vi "Topo & GridSpectr_DriftCorrection_zSpec_v15.vi"(6 "Internal use":string, 7 "Grid param":T1 {"height (m)" format="%#_6p"; "width (m)" format="%#_6p"; "center Y (m)" format="%#_6p"; "center X (m)" format="%#_6p"}, 8 "Error in (no error)":errorcluster, 9 "Points Y/Index Y":i32, 10 "Points X/Index X":i32, 11 "Method":enum16{"init", "run", "end"}(ring)=enum."end") -> (0 "Error out":errorcluster)   [LabVIEW 2014]
doc: "Example of a measurement VI to be used in the \"Experiments on a Grid\" tool as external VI.\n\nThis example measure the topography and spectroscopy data. The spectroscopy measurements are taken on a subgrid. The data are saved to a sxm and a binary file.\n\n- Nanonis Programming Interface -"
uses:
  <userlib>/Nanonis Prog Interface V5/Scan/Grid/GridPatternGet.vi
  <userlib>/Nanonis Prog Interface V5/Scan/Grid/LinePatternGet.vi
  <userlib>/Nanonis Prog Interface V5/Nanonis Prog Interface.lvlib
panel:
  in  "trigger 2 >Hz":sgl format="%#_6p"
  in  "trigger1 < Hz":sgl format="%#_6p"
  out "zFile":refnum<file>
  out "last z adjustment":sgl format="%#_6p"
  in  "during Spec Bias (V)":sgl format="%#_5p"
  in  "type":u16(ring)=1 items=["Line", "Grid"]
  in  "readjust setpoint every":i32=4
  in  "Correct Drift":bool=TRUE
  in  "Email when finished":string="cornelius.krull@monash.edu"
  in  "STS z offset":dbl format="%#_6p"
  out "ETA":timestamp
  out "remaining":dbl format="%<%H:%M:%S>t"
  out "Progress":u8(slide) scale=0.0..100.0 scale format="%#.1g"
  out "total Points":i32
  in  "preSTS delay [ms]":u32=500
  in  "ref Bias":dbl=0.02 format="%#_6p"
  in  "Imaging Bias":dbl=0.02 format="%#_6p"
  in  "max applied Drift Correction":i32=20 min=1 max=100 step=1 format="%.0p"
  in  "Correlate":u16(ring) items=["first Frame", "successive Frames"]
  out "Topo Images taken":i32=14
  in  "Increment":i32=40
  in  "Threshold":i32=2 min=1 step=1
  in  "tip Speed (m/s)":sgl=2e-09 format="%.2p"
  out "X drift":i32
  out "Y drift":i32
  out "Last Drift detected":i32=40
  in  "MaxImagesBack":i32=40
  in  "Channel index (0-23)":u8(ring) items=["Current"=0, "Z (m)"=14]
  in  "File name":string="symmetric_node"
  in  "ref Current":dbl=5e-12 format="%#_6p"
  in  "Imaging Current":dbl=5e-12 format="%#_6p"
  in  "zdrift \nDuration (s)":dbl
  in  "Correct z drift":bool
  out "Status":string="finishing"
  in  "Drift correction Pixels":i32=256 caption="Topo Pixels"
  out "Y Offset":dbl format="%#_6p"
  out "X Offset":dbl format="%#_6p"
  out "Points taken":dbl=14.0
  in  "Drift Correction every":i32=40
  in  "Y subgrid spacing":u16=1
  in  "X subgrid spacing":u16=1
  # "z Spectroscopy"
  # "GRID points"
  # "Increase this if no Drift was detected for \na certain number of images"
  # "%"
  # "time (HH:MM:SS)"
  # "images back"
  # "% of image size"
  # "RUN smart tilt before starting the GRID\nImg Angle = 0\nmove tip to reference point for tip height"
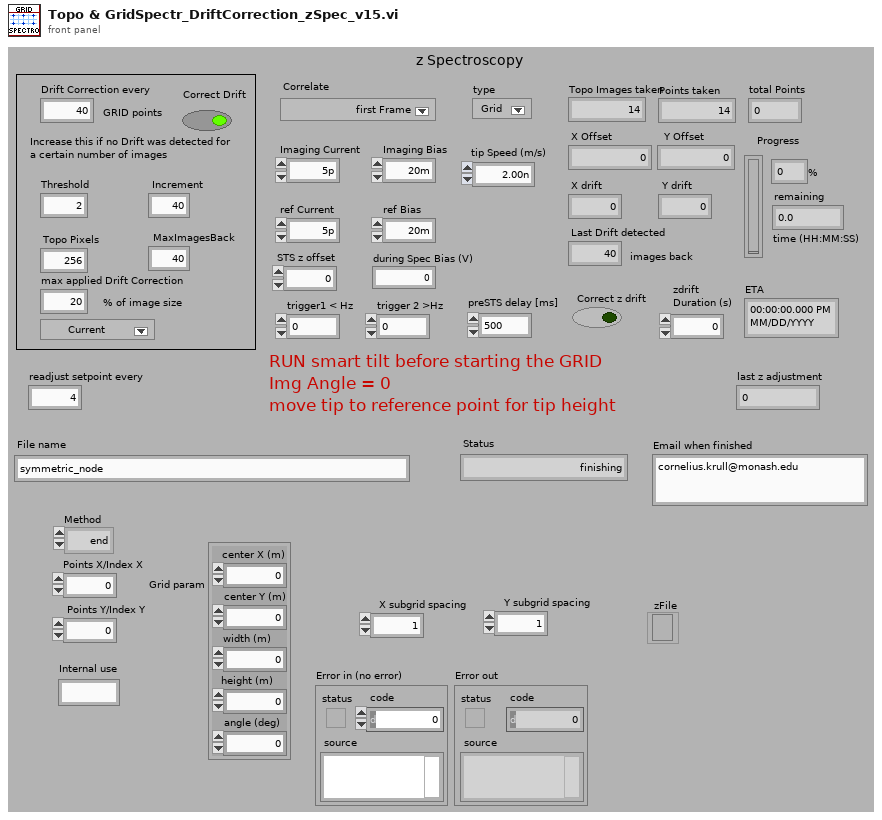
[diagram p1: front panel]
types:
  T1 = cluster{"center X (m)":sgl, "center Y (m)":sgl, "width (m)":sgl, "height (m)":sgl, "angle (deg)":sgl}
  T2 = enum16{"open", "replace", "create", "open or create", "replace or create", "replace or create with confirmation"}
  T3 = cluster{"Z averaging time (s)":sgl, "Z offset (m)":sgl, "Initial settling time (s)":sgl}
  T4 = cluster{"Drift correction Pixels":i32, "Imaging Current":dbl, "STS Current":dbl, "MaxImagesBack":i32, "tip Speed (m/s)":sgl, "Threshold":i32, "Increment":i32, "Correlate":u16, "max applied Drift Correction":i32, "Imaging Bias":dbl, "Move Current":dbl, "Move Bias":dbl, "STS Bias":dbl, "preSTS delay [ms]":u32, "STS z offset":dbl, "Correct Drift":bool, "Lockin ON/OFF":bool}
  T5 = cluster{"center X":sgl, "center Y":sgl, "angle":sgl, "width":sgl, "height":sgl, "# pixels":i32, "# lines":i32}
  T6 = cluster{"Name":string, "Calibration":sgl, "Offset":sgl, "Channel index":i32}[]
  T7 = cluster{"up/down":bool, "time/line":sgl, "start time":timestamp, "end time":timestamp}
  T8 = cluster{"Z averaging time (s)":sgl, "Initial settling time (s)":sgl}
  T9 = cluster{"Max. slew rate (m/s)":sgl, "Settling time (s)":sgl, "Integration time (s)":sgl}
  T10 = cluster{"End settling time (s)":sgl, "Z control time (s)":sgl}
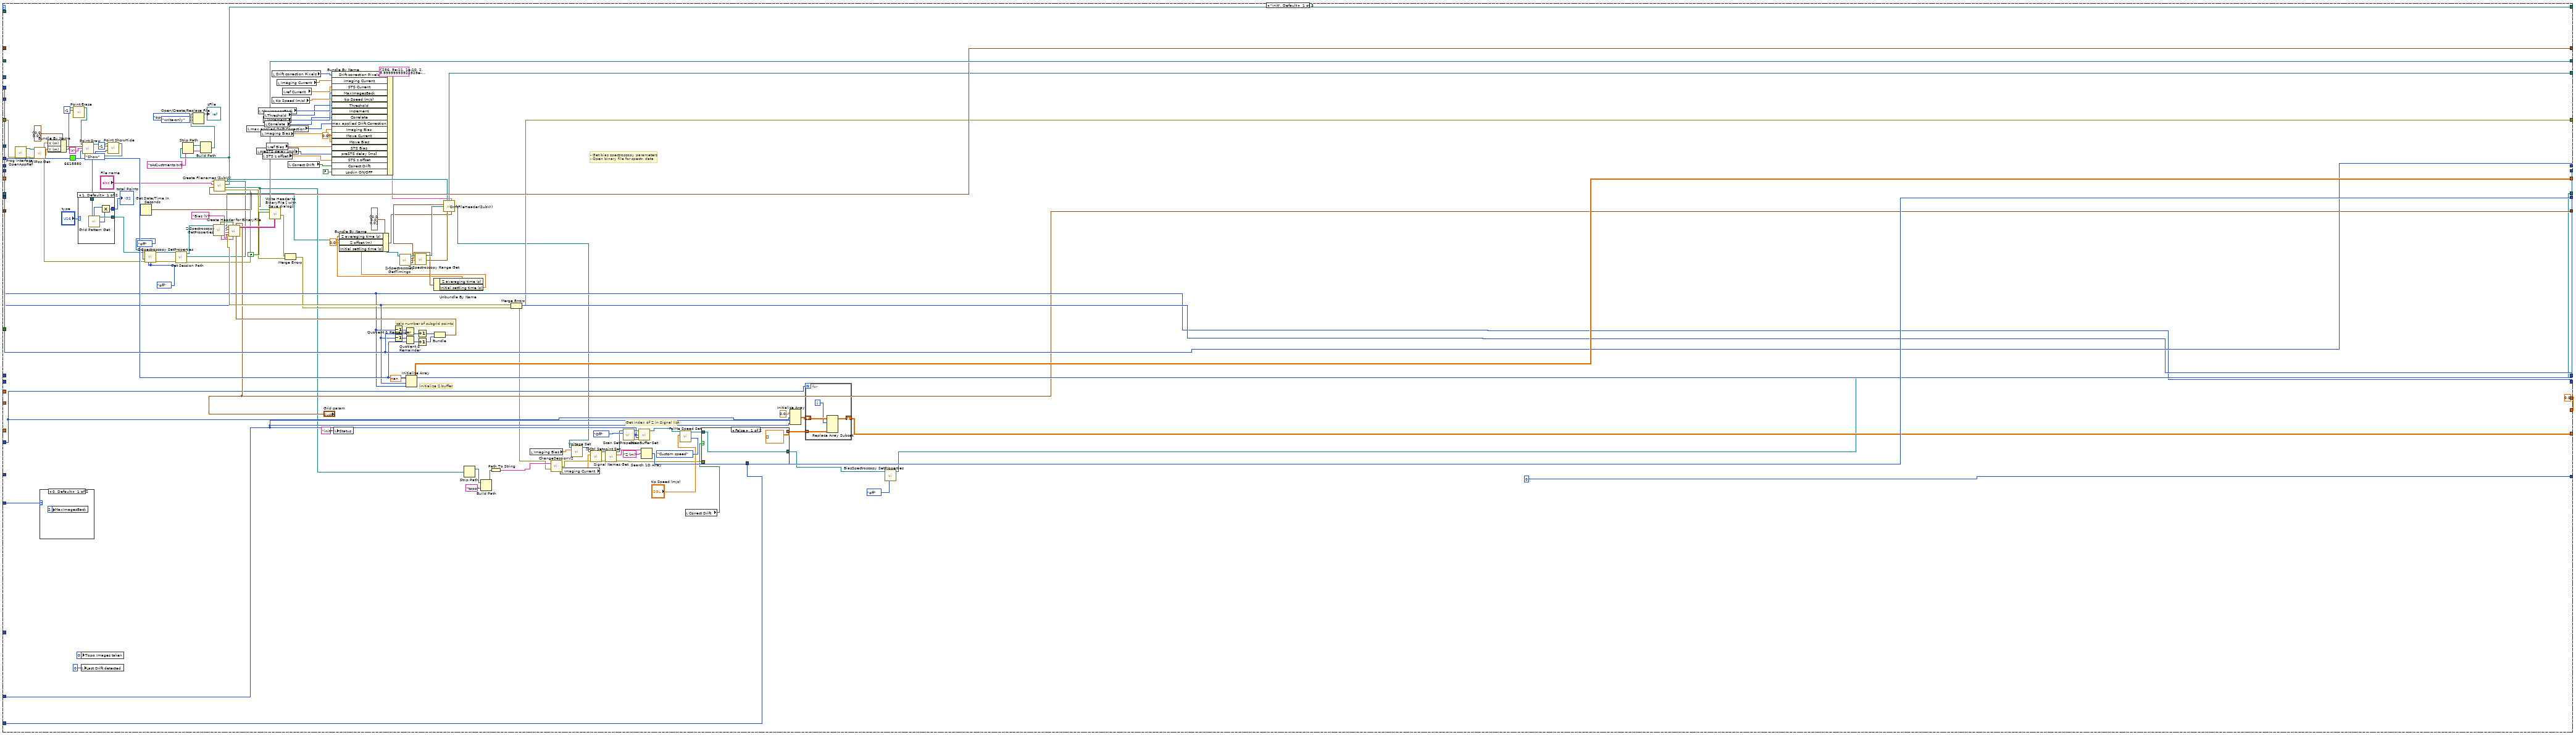
[diagram p2: hidden frame]
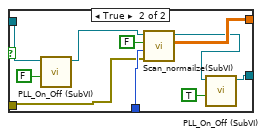
[diagram p3: hidden frame]
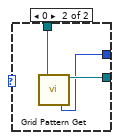
[diagram p4: hidden frame]
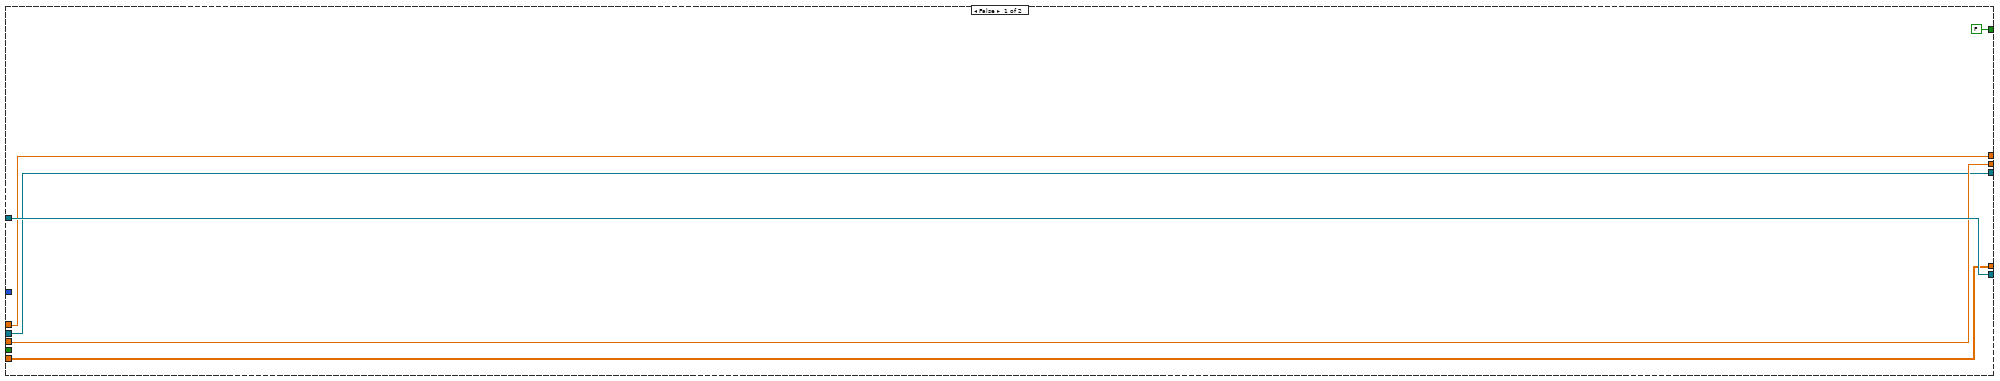
[diagram p9: hidden frame]
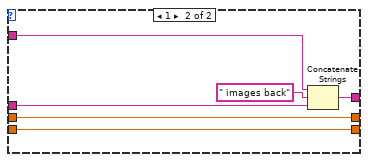
[diagram p10: hidden frame]
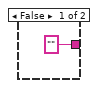
[diagram p12: hidden frame]
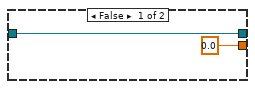
[diagram p13: hidden frame]
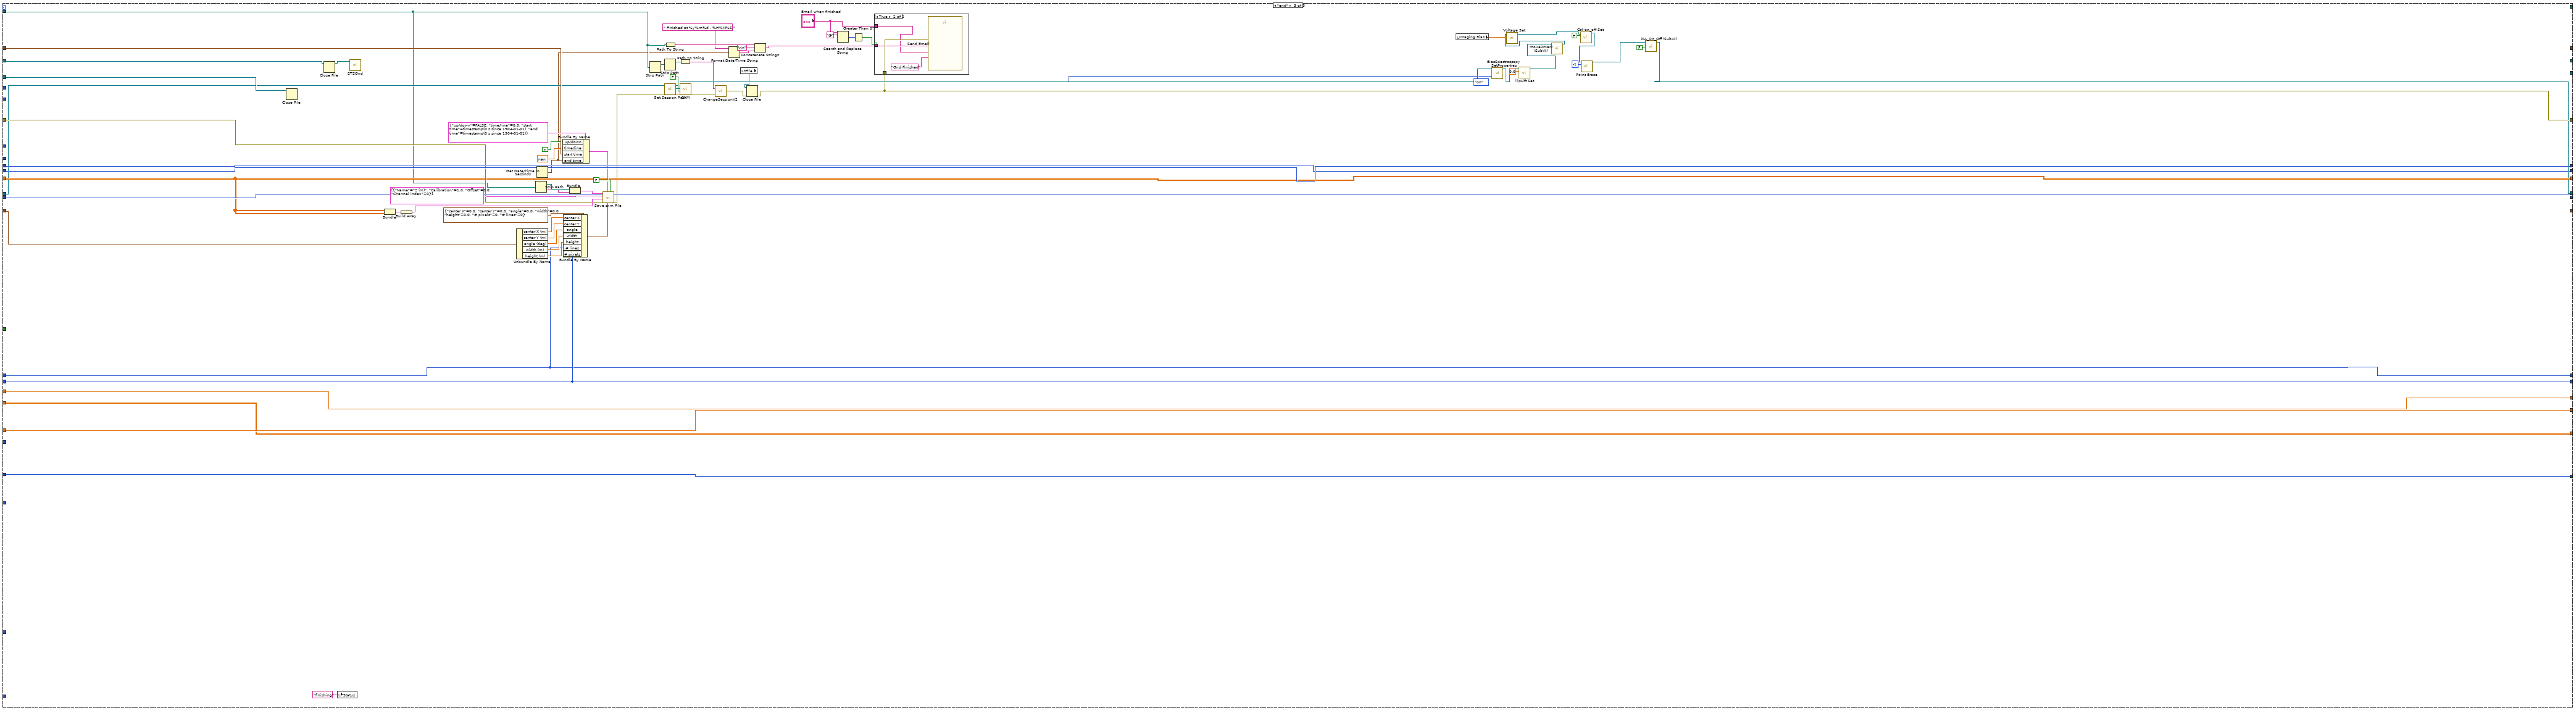
[diagram p15: hidden frame]
diagram:
  # "This string control is required so this VI's connector is compatible with the Nanonis module : \"Experiment on a grid\"."
  # "IMPORTANT : The connector of your own VI must EXACTLY match the connector of this example VI.\n\nThis example VI will do the following:\n- init: Open/Create a sxm (scan data file). Store file path in shift register. Initialize buffer for the topography data. Open binary file and create header.\n- run: Get Z position and write it to topography buffer (from last row to first row of buffer, to make it compatible to Save sxm File function which assumes data starting on the top left corner of image). If grid indices x,y are multiples of the subgrid spacings, start a bias spectroscopy experiment. Write the spectroscopy data to the binary file.\n- end: Write data from topography buffer to file, along with grid dimensions and other known parameters. Close files."
  n1 = while {
    shift-right: [w21] -> _
    shift-left: _ -> [w44]
    shift-right: [w39] -> _
    shift-left: _ -> [w38]
    shift-right: [w36] -> _
    shift-left: _ -> [w37]
    shift-right: [w35] -> _
    shift-left: _ -> [w34]
    shift-right: [w28] -> _
    shift-left: _ -> [w30]
    shift-right: [w29] -> _
    shift-left: _ -> [w31]
    shift-right: [w27] -> _
    shift-left: _ -> [w26]
    shift-right: [w25] -> _
    shift-left: _ -> [w24]
    shift-right: [w23] -> _
    shift-left: _ -> [w22]
    shift-right: [w20] -> _
    shift-left: _ -> [w19]
    shift-right: [w18] -> _
    shift-left: _ -> [w17]
    shift-right: [w16] -> _
    shift-left: _ -> [w9]
    shift-right: [w15] -> _
    shift-left: _ -> [w8]
    shift-right: [w14] -> _
    shift-left: _ -> [w11]
    shift-right: [w13] -> _
    shift-left: _ -> [w10]
    shift-right: [w6] -> _
    shift-left: _ -> [w5]
    stop <- TRUE stop-if-true
    # "> Drift file ref >"
    # "> number of  points  >"
    # "> Ref Frame  >"
    # "> Grid param >"
    # "> start time >"
    # ">Application reference >"
    # "> Y Subgrid spacing >"
    # "> X Subgrid spacing >"
    # "> Z signal index >"
    # "> Binary file ref >"
    # "> Z buffer >"
    # "> sxm file path >"
    n2 = case shown="\"run\"" "Method" {
      tunnel: [w53 w279 _] -> w21
      tunnel: w44 -> [_ w279 w485]
      tunnel: "Error in (no error)" -> [w147 w265 w515]
      tunnel: [w127 w278 w462] -> w42
      tunnel: "Points X/Index X" -> [w159 w273 _]
      tunnel: "Points Y/Index Y" -> [w160 w259 _]
      tunnel: [w183 w276 w504] -> w39
      tunnel: w38 -> [_ w277 w504]
      tunnel: w37 -> [_ w275 w497]
      tunnel: [w175 w274 _] -> w36
      tunnel: [w173 w209 w529] -> w35
      tunnel: w34 -> [_ w209 w529]
      tunnel: "X subgrid spacing" -> [w172 _ _]
      tunnel: "Y subgrid spacing" -> [w171 _ _]
      tunnel: w31 -> [_ w267 w528]
      tunnel: w30 -> [_ w266 w527]
      tunnel: [w172 w267 w528] -> w29
      tunnel: [w171 w266 w527] -> w28
      tunnel: [w112 w252 w460] -> w27
      tunnel: w26 -> [_ w236 w490]
      tunnel: ["Grid param" w262 _] -> w25
      tunnel: w24 -> [_ w262 w514]
      tunnel: [w145 w227 _] -> w23
      tunnel: w22 -> [_ w227 w522]
      tunnel: [w160 w260 w505] -> w20
      tunnel: w19 -> [_ w260 w505]
      tunnel: [w159 w261 w506] -> w18
      tunnel: w17 -> [_ w261 w506]
      tunnel: [w156 w242 w503] -> w16
      tunnel: [w156 w247 w501] -> w15
      tunnel: [w141 w241 w498] -> w14
      tunnel: [0 w225 w502] -> w13
      tunnel: w10 -> [_ w211 w502]
      tunnel: "Drift Correction every" -> [_ w255 _]
      tunnel: w11 -> [_ w246 w498]
      tunnel: w9 -> [_ w253 w503]
      tunnel: w8 -> [_ w239 w501]
      tunnel: "Drift correction Pixels" -> [w140 _ _]
      tunnel: [w108 w244 _] -> w6
      tunnel: w5 -> [_ w245 w499]
      tunnel: "Correct z drift" -> [_ w243 _]
      tunnel: "Channel index (0-23)" -> [w90 w240 _]
      tunnel: "MaxImagesBack" -> [w139 _ _]
      tunnel: "Correlate" -> [w120 _ _]
      frame "init", Default {
        w55 = 0.0 ("Move Current")
        w110 = enum16{"no change", "on", "off"}."off" ("Save dialog")
        w156 = 0.0
        # "- Get bias spectroscopy parameters\n- Open binary file for spectr. data"
        # "initialize Z buffer"
        # "calc number of subgrid points"
        # "Get index of Z in Signal list"
        n3 = call <userlib>:"Prog Interface - OpenAppRef.vi"("Error in (no error)"=w147) -> ("Error out"=w85:errorcluster, "Application reference"=w87:refnum<vi>)  [unwired: 5 in]
        n4 = call <userlib>:"XY-Pos Get.vi"("error in (no error)"=w85, "Application ref in"=w87) -> ("error out"=w86:errorcluster, "Y (m)"=w79:sgl, "X (m)"=w80:sgl, "Application ref out"=w61:refnum<vi>)  [unwired: 5 in]
        n5 = case shown="0, Default" w120 {
          frame 0, Default {
            n6 = local write "MaxImagesBack"(2 ("StepsBack")) -> ()
          }
          frame 1 {
          }
        }
        n7 = Bundle By Name(cluster=cluster{"X (m)":sgl, "Y (m)":sgl} {"X (m)"=0.0, "Y (m)"=0.0} ("Point Coordinates"), "X (m)"=w80, "Y (m)"=w79) -> (w81:cluster{"X (m)":sgl, "Y (m)":sgl})
        n8 = call <userlib>:"Point Erase.vi"("Application ref in"=w61, "Point index (-1=All points)"=-1) -> ("Application ref out"=w60:refnum<vi>)  [unwired: 12 in, 1 out]
        n9 = local write "Topo Images taken"(0 ("Images taken")) -> ()
        n10 = local write "Last Drift detected"(0 ("Last Drift detected")) -> ()
        n11 = call <userlib>:"Point Draw.vi"("Application ref in"=w60, "Point Coordinates"=w81, "Text"="X", "Color"=u32 6618880) -> ("Application ref out"=w65:refnum<vi>)  [unwired: 10 in, 1 out]
        n12 = call <userlib>:"Point ShowHide.vi"("Application ref in"=w65, "Point index (-1=All points)"=-1, "Show/Hide"=enum16{"Show", "Hide"}."Show") -> ("Application ref out"=w64:refnum<vi>)  [unwired: 11 in, 1 out]
        n13 = case shown="1, Default" "type" {
          tunnel: [w200 w203] -> w114
          tunnel: [w197 w201] -> w113
          tunnel: w64 -> [w196 w202]
          frame 1, Default {
            n14 = call-poly <userlib>:"Grid Pattern Get.vi"("Application ref in"=w196) -> ("Points Y"=w198:i32, "Points X"=w199:i32, "Application ref out"=w200:refnum<vi>)  [unwired: 10 in, 6 out]
            n15 = Multiply(x=w198, y=w199) -> (x*y=w197:i32)
          }
          frame 0 {
            n16 = call-poly <userlib>:"Grid Pattern Get.vi"("Application ref in"=w202) -> ("Points"=w201:i32, "Application ref out"=w203:refnum<vi>)  [unwired: 12 in, 5 out]
          }
        }
        "total Points" <- w113
        n17 = Get Date/Time In Seconds() -> (seconds since 1Jan1904=w145:timestamp)
        n18 = call <userlib>:"Z-Spectroscopy SetProperties.vi"("Application ref in"=w114, "Autosave"=enum16{"no change", "on", "off"}."off" ("Autosave (no change)"), "error in (no error)"=w86, "Save dialog"=w110, "Save all sweeps (no change)"=w110) -> ("Application ref out"=w123:refnum<vi>, "error out"=w122:errorcluster)  [unwired: 9 in]
        n19 = call <userlib>:"Get Session Path.vi"("error in (no error)"=w122, "Application ref in"=w123) -> ("error out"=w146:errorcluster, "Session path"=w133:path, "Application ref out"=w124:refnum<vi>)  [unwired: 7 in]
        n20 = call <userlib>:"Z-Spectroscopy GetProperties.vi"("Application ref in"=w124) -> ("Backward sweep"=w179:bool, "Application ref out"=w76:refnum<vi>, "Number of points"=w162:i32, "Channels"=w161:string[], "Parameters"=w177:string[], "Fixed parameters"=w164:string[], "error out"=w176:errorcluster)  [unwired: 7 in, 1 out]
        n21 = call "Create Filenames (SubVI).vi"("error in (no error)"=w146, "seconds since 1Jan1904"=w145, "File name"="File name", "Session path"=w133) -> ("error out"=w136:errorcluster, "binFilePath"=w129:path, "topoFilePath"=w53:path, "Drift File out"=w109:refnum<file>)  [unwired: 4 in]
        n22 = Strip Path(path=w53) -> (stripped path=w52:path)  [unwired: 1 out]
        n23 = Build Path(base path=w52, name or relative path="zAdjustments.txt") -> (appended path=w50:path)
        n24 = Open/Create/Replace File(file path (use dialog)=w50, operation (0:open)=T2."open or create", access (0:read/write)=enum16{"read/write", "read-only", "write-only"}."write-only") -> (refnum out=→"zFile":refnum<file>)  [unwired: 3 in, 2 out]
        n25 = local read "max applied Drift Correction"() -> (w96:i32)
        n26 = local read "preSTS delay [ms]"() -> (w93:u32)
        n27 = local read "MaxImagesBack"() -> (w100:i32)
        n28 = local read "Imaging Bias"() -> (w95:dbl)
        n29 = local read "STS z offset"() -> (w92:dbl)
        n30 = local read "Increment"() -> (w98:i32)
        n31 = local read "Threshold"() -> (w99:i32)
        n32 = local read "Correlate"() -> (w97:u16)
        n33 = local read "ref Bias"() -> (w94:dbl)
        n34 = local read "Drift correction Pixels"() -> (w104:i32)
        n35 = local read "tip Speed (m/s)"() -> (w101:sgl)
        n36 = local read "Imaging Current"() -> (w103:dbl)
        n37 = local read "ref Current"() -> (w102:dbl)
        n38 = local read "Correct Drift"() -> (w91:bool)
        n39 = Bundle By Name(cluster=T4 {"Drift correction Pixels"=256, "Imaging Current"=5e-11, "STS Current"=1e-10, "MaxImagesBack"=2, "tip Speed (m/s)"=1e-08, "Threshold"=2, "Increment"=64, "Correlate"=0, "max applied Drift Correction"=20, "Imaging Bias"=-0.02, "Move Current"=1.5e-11, "Move Bias"=-0.02, "STS Bias"=0.1, "preSTS delay [ms]"=1000, "STS z offset"=-1.7e-10, "Correct Drift"=TRUE, "Lockin ON/OFF"=TRUE} ("Drift Correction"), "Drift correction Pixels"=w104, "Imaging Current"=w103, "STS Current"=w102, "MaxImagesBack"=w100, "tip Speed (m/s)"=w101, "Threshold"=w99, "Increment"=w98, "Correlate"=w97, "max applied Drift Correction"=w96, "Imaging Bias"=w95, "Move Current"=w55, "Move Bias"=w55, "STS Bias"=w94, "preSTS delay [ms]"=w93, "STS z offset"=w92, "Correct Drift"=w91, "Lockin ON/OFF"=FALSE) -> (w106:T4)
        n40 = local write "Status"("init" ("Status")) -> ()
        n41 = Decrement(x=w159) -> (x-1=w170:i32)
        n42 = Decrement(x=w160) -> (x-1=w169:i32)
        n43 = call <userlib>:"Z-Spectroscopy GetTimings.vi"("Application ref in"=w76) -> ("Application ref out"=w77:refnum<vi>, "Initialization"=w72:T8, "Sweep Timing"=w73:T9, "End of Sweep"=w74:T10, "Error out"=w78:errorcluster)  [unwired: 10 in]
        n44 = Quotient & Remainder(x=w170, y=w172) -> (floor(x/y)=w168:i32)  [unwired: 1 out]
        n45 = Quotient & Remainder(x=w169, y=w171) -> (floor(x/y)=w167:i32)  [unwired: 1 out]
        n46 = Initialize Array(sgl nan ("element"), w160, w159) -> (w183:sgl[][])
        n47 = call <userlib>:"Z-Spectroscopy Range Get.vi"("error in (no error)"=w78, "Application ref in"=w77) -> ("Application ref out"=w75:refnum<vi>)  [unwired: 5 in, 3 out]
        n48 = Increment(x=w168) -> (x+1=w166:i32)
        n49 = Increment(x=w167) -> (x+1=w165:i32)
        n50 = Unbundle By Name(w72) -> ("Z averaging time (s)"=w69:sgl, "Initial settling time (s)"=w68:sgl)
        n51 = Bundle By Name(cluster=T3 {"Z averaging time (s)"=0.0, "Z offset (m)"=0.0, "Initial settling time (s)"=0.0} ("Initialization"), "Z averaging time (s)"=w69, "Z offset (m)"=sgl 0.0, "Initial settling time (s)"=w68) -> (w70:T3)
        n52 = Bundle(w166, w165) -> (w178:cluster{i32, i32})  [unwired: 1 in]
        n53 = call <userlib>:"Create Header for BinaryFile.vi"("Grid points"=w178, "Grid param"="Grid param", "Fixed parameters"=w164, "Backward sweep"=w179, "Sweep signal"="Bias (V)" ("Sweep Signal"), "Parameters"=w177, "Channels"=w161, "Points per sweep"=w162) -> ("Header (fixed attributes)"=w181:string[][])  [unwired: 3 in]
        n54 = call <userlib>:"Write Header to BinaryFile [ with Save dialog].vi"("Fixed Attributes"=w181, "Show Dialog? (T)"=FALSE, "Filename"=w129) -> ("Error out"=w137:errorcluster, "File ref"=w175:refnum<file>)  [unwired: 5 in, 2 out]
        n55 = Merge Errors(w137, w136) -> (w138:errorcluster)
        n56 = call "DriftFileHeader(SubVI).vi"("Byte Stream File in"=w109, "Drift Correction"=w106, "End of Sweep"=w74, "Application ref in"=w75, "Sweep Timing"=w73, "Initialization"=w70) -> ("Byte Stream File out"=w108:refnum<file>, "Application ref out"=w107:refnum<vi>)  [unwired: 8 in]
        n57 = Strip Path(path=w129) -> (stripped path=w132:path)  [unwired: 1 out]
        n58 = Build Path(base path=w132, name or relative path="topo") -> (appended path=w130:path)
        n59 = Path To String(path=w130) -> (string=w128:string)
        n60 = Merge Errors(w176, w138) -> (w127:errorcluster)
        n61 = local read "Imaging Bias"() -> (w116:dbl)
        n62 = call "ChangeSessionV2.vi"("error in (no error)"=w127, "Session"=w128) -> ("error out"=w126:errorcluster)
        n63 = local read "Imaging Current"() -> (w115:dbl)
        n64 = call <userlib>:"Voltage Set.vi"("Bias (V)"=w116, "Application ref in"=w107) -> ("Application ref out"=w117:refnum<vi>)  [unwired: 8 in, 1 out]
        n65 = call <userlib>:"Z-Ctrl Setpoint Set.vi"("error in (no error)"=w126, "Z Controller setpoint"=w115, "Application ref in"=w117) -> ("error out"=w148:errorcluster, "Application ref out"=w149:refnum<vi>)  [unwired: 7 in]
        n66 = call <userlib>:"Signal Names Get.vi"("error in (no error)"=w148, "Application ref in"=w149) -> ("error out"=w89:errorcluster, "Signals Names"=w163:string[], "Application ref out"=w152:refnum<vi>)  [unwired: 5 in]
        n67 = call <userlib>:"Scan SetProperties.vi"("Application ref in"=w152, "Continuous scan"=enum16{"No change", "On", "Off"}."Off") -> ("Application ref out"=w154:refnum<vi>, "Error out"=w153:errorcluster)  [unwired: 12 in]
        n68 = call <userlib>:"ScanBuffer Set.vi"("Application ref in"=w154, "Pixels"=w140, "Lines"=w140, "error in (no error)"=w153) -> ("Application ref out"=w118:refnum<vi>)  [unwired: 10 in, 1 out]
        n69 = Search 1D Array(1D array=w163, element="Z (m)") -> (index of element=w173:i32)  [unwired: 1 in]
        n70 = call <userlib>:"FolMe Speed Set.vi"("Speed Setting (Custom)"=enum32{"Scan speed", "Custom speed"}."Custom speed", "Speed (m/s)"="tip Speed (m/s)", "Application ref in"=w118) -> ("Application ref out"=w58:refnum<vi>)  [unwired: 5 in, 1 out]
        n71 = local read "Correct Drift"() -> (w56:bool)
        n72 = case shown="False" w56 {
          tunnel: w90 -> [_ w195]
          tunnel: w89 -> [_ w194]
          tunnel: [dbl[][] [] ("Array") w193] -> w88
          tunnel: w58 -> [w185 w191]
          tunnel: [w185 w186] -> w54
          frame False {
          }
          frame True {
            n73 = call "PLL_On_Off (SubVI).vi"("Output ON/OFF (F=OFF)"=FALSE, "Application in"=w191) -> ("Application out"=w190:refnum<vi>)  [unwired: 8 in, 1 out]
            n74 = call "Scan_normailze(SubVI).vi"("error in (no error)"=w194, "Channel index (0-23)"=w195, "Normalization"=FALSE ("Boolean"), "Application in"=w190) -> ("Array"=w193:dbl[][], "Application out"=w187:refnum<vi>)  [unwired: 5 in, 1 out]
            n75 = call "PLL_On_Off (SubVI).vi"("Output ON/OFF (F=OFF)"=TRUE, "Application in"=w187) -> ("Application out"=w186:refnum<vi>)  [unwired: 8 in, 1 out]
          }
        }
        n76 = Initialize Array(0.0 ("element"), w139, w140, w140) -> (w142:dbl[][][])
        n77 = for {
          N: w139 -> [_]
          tunnel: w88 -> [w207]
          shift-right: [w206] -> w141
          shift-left: w142 -> [w208]
          i -> [w205]
          n78 = Replace Array Subset(array=w208, new element=w207, index (dim 0)=w205) -> (w206:dbl[][][])  [unwired: 2 in]
        }
        n79 = call <userlib>:"BiasSpectroscopy SetProperties.vi"("Application ref in"=w54, "Z-Controller hold (no change)"=enum16{"no change", "on", "off"}."off") -> ("Application ref out"=w112:refnum<vi>)  [unwired: 12 in, 1 out]
      }
      frame "run" {
        # "shift tip position"
        # "Get Z position"
        # "- get Z position for topography and store it to Z buffer\n- if x,y indices are a multiple of the spacings, take spectroscopy curve and write data to binary file\ndo drift correction if number of STS position was reached"
        n80 = local read "Correct Drift"() -> (w219:bool)
        n81 = Quotient & Remainder(x=w211, y=w255) -> (x-y*floor(x/y)=w256:i32)  [unwired: 1 out]
        n82 = Not Equal To 0?(x=w211) -> (x != 0?=w237:bool)
        n83 = Equal To 0?(x=w256) -> (x = 0?=w254:bool)
        n84 = call <userlib>:"XY-Pos Get.vi"("Wait for newest data (F=False)"=TRUE, "Application ref in"=w236) -> ("Y (m)"=w232:sgl, "X (m)"=w233:sgl, "Application ref out"=w235:refnum<vi>)  [unwired: 5 in, 1 out]
        n85 = Compound Arithmetic op=AND(w237, w254, w219) -> (w238:bool)
        n86 = case shown="True" w238 {
          tunnel: w235 -> [w340 w352]
          tunnel: [w340 w397] -> w216
          tunnel: w246 -> [w337 w393]
          tunnel: [w339 w395] -> w242
          tunnel: [w338 w394] -> w247
          tunnel: w253 -> [w339 w376]
          tunnel: w239 -> [w338 w374]
          tunnel: [w337 w389] -> w241
          tunnel: w245 -> [w336 w400]
          tunnel: [w336 w399] -> w244
          tunnel: w243 -> [_ w396]
          tunnel: w240 -> [_ w380]
          tunnel: [FALSE TRUE] -> w213
          frame False {
          }
          frame True {
            # "Drift correction \ncompare to the reference image with the previous image \ndx and dy will be applied to the grid coord, \nand the imaging frame will be shifted"
            n87 = Greater Or Equal To 0?(x=w380) -> (x >= 0?=w379:bool)
            n88 = call "move2mark (SubVI).vi"("Application in"=w352) -> ("Application out"=w351:refnum<vi>)  [unwired: 10 in]
            n89 = local write "Status"("Drift Correction" ("Status")) -> ()
            n90 = case shown="True" w379 {
              frame False {
              }
              frame True {
                n91 = local read "Topo Images taken"() -> (w415:i32)
                n92 = Increment(x=w415) -> (x+1=w414:i32)
                n93 = local write "Topo Images taken"(w414) -> ()
              }
            }
            n94 = local read "Imaging Bias"() -> (w359:dbl)
            n95 = call <userlib>:"Voltage Set.vi"("Bias (V)"=w359, "Application ref in"=w351) -> ("Application ref out"=w360:refnum<vi>)  [unwired: 8 in, 1 out]
            n96 = local read "Imaging Current"() -> (w358:dbl)
            n97 = call <userlib>:"Z-Ctrl Setpoint Set.vi"("Z Controller setpoint"=w358, "Application ref in"=w360) -> ("Application ref out"=w350:refnum<vi>)  [unwired: 8 in, 1 out]
            n98 = call <userlib>:"Ctrl-on_off Set.vi"("Z Controller ON/OFF"=TRUE, "Application ref in"=w350) -> ("Application ref out"=w348:refnum<vi>)  [unwired: 8 in, 1 out]
            n99 = call "PLL_On_Off (SubVI).vi"("Output ON/OFF (F=OFF)"=FALSE, "Application in"=w348) -> ("Application out"=w347:refnum<vi>)  [unwired: 8 in, 1 out]
            n100 = call "Scan_normailze(SubVI).vi"("Channel index (0-23)"=w380, "Normalization"=FALSE ("Boolean"), "Application in"=w347) -> ("Array"=w390:dbl[][], "Application out"=w345:refnum<vi>)  [unwired: 6 in, 1 out]
            n101 = Divide(x="max applied Drift Correction", y=100) -> (x/y=w367:dbl)
            n102 = local read "Drift correction Pixels"() -> (w368:i32)
            n103 = local read "Last Drift detected"() -> (w371:i32)
            n104 = local read "Correlate"() -> (w377:u16)
            n105 = call "PLL_On_Off (SubVI).vi"("Output ON/OFF (F=OFF)"=TRUE, "Application in"=w345) -> ("Application out"=w342:refnum<vi>)  [unwired: 8 in, 1 out]
            n106 = Multiply(x=w367, y=w368) -> (x*y=w369:dbl)
            n107 = call "CorrelImages (SubVI)v2.vi"("last drift detected"=w371, "Correlate"=w377, "Ref Array"=w393, "New Image"=w390) -> ("Y drift"=w365:i32, "X drift"=w362:i32, "Ref Array out"=w389:dbl[][][], "Queue Steps"=w378:i32)  [unwired: 4 in]
            "X drift" <- w362
            "Y drift" <- w365
            "Last Drift detected" <- w378
            n108 = local read "Topo Images taken"() -> (w382:i32)
            n109 = To Long Integer(number=w369) -> (32bit integer=w361:i32)
            n110 = Greater Or Equal?(x=w378, y="Threshold") -> (x >= y?=w384:bool)
            n111 = Greater?(x=w382, y="Threshold") -> (0:w381:bool)
            n112 = call "AbsLimit (SubVI).vi"("in"=w362, "Abslimt"=w361) -> ("Numeric out"=w364:i32)  [unwired: 9 in]
            n113 = call "AbsLimit (SubVI).vi"("in"=w365, "Abslimt"=w361) -> ("Numeric out"=w363:i32)  [unwired: 9 in]
            n114 = And(x=w384, y=w381) -> (x .and. y?=w383:bool)
            n115 = case shown="True" w383 {
              tunnel: ["" w419] -> w385
              frame False {
              }
              frame True {
                n116 = local read "Drift Correction every"() -> (w418:i32)
                n117 = local write "Last Drift detected"(0 ("Last Drift detected")) -> ()
                n118 = Add(x=w418, y="Increment") -> (x+y=w422:i32)
                n119 = local write "Drift Correction every"(w422) -> ()
                n120 = Number To Decimal String(number=w422) -> (decimal integer string=w421:string)  [unwired: 1 in]
                n121 = Concatenate Strings(" Increased DC to every " ("string"), w421) -> (w419:string)
              }
            }
            n122 = local read "Drift correction Pixels"() -> (w387:i32)
            n123 = Number To Decimal String(number=w378) -> (decimal integer string=w392:string)  [unwired: 1 in]
            n124 = case shown="0, Default" w377 {
              tunnel: w392 -> [w402 w413]
              tunnel: [w407 w412] -> w391
              tunnel: w385 -> [w405 w410]
              tunnel: w376 -> [w403 w409]
              tunnel: [w403 w409] -> w375
              tunnel: w374 -> [w404 w408]
              tunnel: [w404 w408] -> w373
              frame 0, Default {
                n125 = Concatenate Strings(w402, "images back , Correlating first frame " ("string"), w405) -> (w407:string)
              }
              frame 1 {
                n126 = Concatenate Strings(w413, " images back" ("string"), w410) -> (w412:string)
              }
            }
            n127 = call "drift_pixel2m (SubVI).vi"("Application in"=w342, "X drift"=w364, "Y drift"=w363, "Drift correction Pixels"=w387) -> ("Application out"=w386:refnum<vi>, "x drift"=w356:sgl, "y drift"=w355:sgl)  [unwired: 2 in, 1 out]
            n128 = local read "type"() -> (w341:u16)
            n129 = call "ShiftFrame (SubVI).vi"("Y shift"=w355, "X shift"=w356, "Application in"=w386) -> ("Application out"=w388:refnum<vi>)  [unwired: 8 in]
            n130 = call "MoveGrid.vi"("type"=w341, "y"=w355, "x"=w356, "Application ref in"=w388) -> ("Application ref out"=w354:refnum<vi>)  [unwired: 6 in, 1 out]
            n131 = call "shift marks (SubVI).vi"("y"=w355, "x"=w356, "Application in"=w354) -> ("Application out"=w353:refnum<vi>)  [unwired: 7 in, 1 out]
            n132 = case shown="True" w396 {
              tunnel: [0.0 ("z drift") w429] -> w398
              tunnel: w353 -> [w424 w428]
              tunnel: [w424 w427] -> w397
              frame False {
              }
              frame True {
                n133 = call "Zdrift_subVi.vi"("Duration"="zdrift \nDuration (s)", "Application in"=w428) -> ("z drift"=w429:dbl, "Application out"=w427:refnum<vi>)  [unwired: 7 in, 1 out]
              }
            }
            n134 = Add(x=w375, y=w356) -> (x+y=w395:dbl)
            n135 = Add(x=w355, y=w373) -> (x+y=w394:dbl)
            n136 = local write "X Offset"(w395) -> ()
            n137 = local write "Y Offset"(w394) -> ()
            n138 = call "Drift Data to file (SubVI).vi"("z drift"=w398, "Comment"=w391, "y Drift"=w394, "X drift"=w395, "Byte Stream File in"=w400) -> ("Byte Stream File out"=w399:refnum<file>)  [unwired: 6 in]
          }
        }
        n139 = Quotient & Remainder(x=w211, y="readjust setpoint every") -> (x-y*floor(x/y)=w212:i32)  [unwired: 1 out]
        n140 = Equal To 0?(x=w211) -> (x = 0?=w210:bool)
        n141 = Equal To 0?(x=w212) -> (x = 0?=w215:bool)
        n142 = Compound Arithmetic op=OR(w210, w213, w215) -> (w214:bool)
        n143 = case shown="True" w214 {
          tunnel: [w280 w297] -> w217
          tunnel: w216 -> [w280 w313]
          tunnel: w209 -> [_ w299]
          frame False {
          }
          frame True {
            n144 = call "move2mark (SubVI).vi"("Application in"=w313) -> ("Application out"=w302:refnum<vi>)  [unwired: 10 in]
            n145 = local write "Status"("adjust setpoint" ("Status")) -> ()
            n146 = local read "ref Bias"() -> (w312:dbl)
            n147 = call <userlib>:"Signal Value Get (Animation period) v2.vi"("Wait for newest data (F=False)"=TRUE, "Signal index (0-79)"=w299, "Application ref in"=w302) -> ("Signal value"=w295:sgl, "Application ref out"=w301:refnum<vi>)  [unwired: 5 in, 1 out]
            n148 = local read "ref Current"() -> (w309:dbl)
            n149 = call <userlib>:"Voltage Set.vi"("Bias (V)"=w312, "Application ref in"=w301) -> ("Application ref out"=w310:refnum<vi>)  [unwired: 8 in, 1 out]
            n150 = flat-sequence {
              tunnel: w310 -> [w318]
              tunnel: [w315] -> w308
              tunnel: w309 -> [w317]
              tunnel: w308 -> [w321]
              tunnel: [w321] -> w307
              tunnel: "preSTS delay [ms]" -> [w319]
              tunnel: w307 -> [w326]
              tunnel: [w323] -> w311
              tunnel: [w324] -> w305
              tunnel: w311 -> [w330]
              tunnel: "preSTS delay [ms]" -> [w329]
              tunnel: w305 -> [_]
              tunnel: [w330] -> w303
              tunnel: [w332] -> w298
              tunnel: w303 -> [w333]
              frame #0 {
                n151 = call <userlib>:"Z-Ctrl Setpoint Set.vi"("Z Controller setpoint"=w317, "Application ref in"=w318) -> ("Application ref out"=w316:refnum<vi>)  [unwired: 8 in, 1 out]
                n152 = call <userlib>:"Ctrl-on_off Set.vi"("Z Controller ON/OFF"=TRUE, "Application ref in"=w316) -> ("Application ref out"=w315:refnum<vi>)  [unwired: 8 in, 1 out]
              }
              frame #1 {
                n153 = Greater Than 0?(x=w319) -> (x > 0?=w320:bool)
                n154 = case shown="True" w320 {
                  tunnel: w319 -> [_ w322]
                  frame False {
                  }
                  frame True {
                    n155 = Wait (ms)(milliseconds to wait=w322) -> ()  [unwired: 1 out]
                  }
                }
              }
              frame #2 {
                n156 = local read "STS z offset"() -> (w324:dbl)
                n157 = call <userlib>:"TipLift Set.vi"("TipLift (m)"=w324, "Application ref in"=w326) -> ("Application ref out"=w325:refnum<vi>)  [unwired: 8 in, 1 out]
                n158 = call <userlib>:"Ctrl-on_off Set.vi"("Z Controller ON/OFF"=FALSE, "Application ref in"=w325) -> ("Application ref out"=w323:refnum<vi>)  [unwired: 8 in, 1 out]
              }
              frame #3 {
                n159 = Greater Than 0?(x=w329) -> (x > 0?=w328:bool)
                n160 = case shown="True" w328 {
                  tunnel: w329 -> [_ w331]
                  frame False {
                  }
                  frame True {
                    n161 = Wait (ms)(milliseconds to wait=w331) -> ()  [unwired: 1 out]
                  }
                }
              }
              frame #4 {
                n162 = call <userlib>:"Voltage Set.vi"("Bias (V)"="during Spec Bias (V)", "Application ref in"=w333) -> ("Application ref out"=w332:refnum<vi>)  [unwired: 8 in, 1 out]
              }
            }
            n163 = Get Date/Time In Seconds() -> (seconds since 1Jan1904=w286:timestamp)
            n164 = Get Date/Time String(date format (0)=enum16{"short", "long", "abbreviated"}."short", seconds (now)=w286, want seconds? (F)=TRUE) -> (date string=w290:string, time string=w289:string)
            n165 = local read "zFile"() -> (w293:refnum<file>)
            n166 = Concatenate Strings(w290, w289, "," ("string")) -> (w288:string)
            n167 = call <userlib>:"Signal Value Get (Animation period) v2.vi"("Wait for newest data (F=False)"=TRUE, "Signal index (0-79)"=w299, "Application ref in"=w298) -> ("Signal value"=w294:sgl, "Application ref out"=w297:refnum<vi>)  [unwired: 5 in, 1 out]
            n168 = Subtract(x=w295, y=w294) -> (x-y=w292:sgl)
            "last z adjustment" <- w292
            n169 = Format Into String(format string="%#g", initial string=w288, w292) -> (resulting string=w283:string)  [unwired: 1 in, 1 out]
            n170 = Concatenate Strings(w283, "\r\n") -> (w282:string)
            n171 = Write to Text File(file (use dialog)=w293, text=w282) -> ()  [unwired: 2 in, 3 out]
          }
        }
        n172 = Quotient & Remainder(x=w273, y=w267) -> (x-y*floor(x/y)=w272:i32)  [unwired: 1 out]
        n173 = Quotient & Remainder(x=w259, y=w266) -> (x-y*floor(x/y)=w271:i32)  [unwired: 1 out]
        n174 = Equal To 0?(x=w272) -> (x = 0?=w270:bool)
        n175 = Equal To 0?(x=w271) -> (x = 0?=w269:bool)
        n176 = And(x=w270, y=w269) -> (x .and. y?=w268:bool)
        n177 = Subtract(x=w260, y=w259) -> (x-y=w258:i32)
        n178 = Decrement(x=w258) -> (x-1=w257:i32)
        n179 = Add(x=w233, y=w242) -> (x+y=w249:dbl)
        n180 = Add(x=w232, y=w247) -> (x+y=w248:dbl)
        n181 = call <userlib>:"XY-Pos Set.vi"("Y (m)"=w248, "X (m)"=w249, "Application ref in"=w217) -> ("Application ref out"=w250:refnum<vi>)  [unwired: 5 in, 1 out]
        n182 = call <userlib>:"Signal Value Get (Animation period).vi"("error in (no error)"=w265, "Signal index (0-47)"=w209, "Application ref in"=w250) -> ("error out"=w264:errorcluster, "Signal value"=w263:sgl, "Application ref out"=w251:refnum<vi>)  [unwired: 5 in]
        n183 = Replace Array Subset(array=w277, new element=w263, index (row)=w257, index (col)=w273) -> (w276:sgl[][])
        n184 = case shown="True" w268 {
          tunnel: [w432 w434] -> w278
          tunnel: w275 -> [w433 w457]
          tunnel: [w433 w455] -> w274
          tunnel: w264 -> [w432 w437]
          tunnel: w251 -> [w431 w440]
          tunnel: [w431 w441] -> w252
          tunnel: [w430 w443] -> w225
          tunnel: w211 -> [w430 w444]
          frame False {
            # "Point indices aren't multiple of subgrid spacing\n=> no spectroscopy at this point"
          }
          frame True {
            # "remove Bias from data"
            n185 = local write "Status"("zSpec" ("Status")) -> ()
            n186 = call "zSpec_trigger.vi"("Error in (no error)"=w437, "trigger 2"="trigger 2 >Hz", "trigger1"="trigger1 < Hz", "Application ref in"=w440) -> ("Error out"=w436:errorcluster)  [unwired: 5 in, 1 out]
            n187 = call <userlib>:"Z-Spectroscopy Start.vi"("Application ref in"=w440, "Get data (F=False)"=TRUE ("Get Data (F)"), "error in (no error)"=w437) -> ("Application ref out"=w441:refnum<vi>, "Data"=w454:sgl[][], "Parameters"=w453:sgl[], "error out"=w446:errorcluster)  [unwired: 8 in, 1 out]
            n188 = Delete From Array(array=w454, length=1, index (row)=0 ("index")) -> (array with subset deleted=w452:sgl[][])  [unwired: 1 in, 1 out]
            n189 = Write to Binary File(file (use dialog)=w457, data=w453, error in=w446, 5:FALSE ("prepend array or string size? (T)")) -> (refnum out=w456:refnum<file>, error out=w445:errorcluster)  [unwired: 2 in, 1 out]
            n190 = Write to Binary File(file (use dialog)=w456, data=w452, error in=w445, 5:FALSE ("prepend array or string size? (T)")) -> (refnum out=w455:refnum<file>, error out=w435:errorcluster)  [unwired: 2 in, 1 out]
            n191 = Increment(x=w444) -> (x+1=w443:i32)
            n192 = Merge Errors(w436, w435) -> (w434:errorcluster)
          }
        }
        n193 = Get Date/Time In Seconds() -> (seconds since 1Jan1904=w222:timestamp)
        n194 = local read "total Points"() -> (w228:i32)
        n195 = Subtract(x=w222, y=w227) -> (x-y=w226:dbl)
        n196 = Divide(x=w225, y=w228) -> (x/y=w231:dbl)
        n197 = Subtract(x=w228, y=w225) -> (x-y=w223:i32)
        n198 = Divide(x=w226, y=w225) -> (x/y=w224:dbl)
        n199 = Multiply(x=w224, y=w223) -> (x*y=w221:dbl)
        "remaining" <- w221
        n200 = Multiply(x=w231, y=100.0) -> (x*y=→"Progress":dbl)
        n201 = Add(x=w222, y=w221) -> (x+y=→"ETA":timestamp)
      }
      frame "end" {
        n202 = Close File(refnum=w499) -> ()  [unwired: 1 in, 2 out]
        n203 = Close File(refnum=w497) -> (path=w496:path)  [unwired: 1 in, 1 out]
        n204 = local write "Status"("finishing" ("Status")) -> ()
        n205 = call "STSGrid.vi"("Binary Spectroscopy File"=w496) -> ()  [unwired: 11 in]
        n206 = Bundle(w504, w504) -> (w526:cluster{sgl[][], sgl[][]})  [unwired: 1 in]
        n207 = Build Array(w526) -> (w525:cluster{sgl[][], sgl[][]}[])
        n208 = Unbundle By Name(w514) -> ("center X (m)"=w512:sgl, "center Y (m)"=w511:sgl, "angle (deg)"=w510:sgl, "width (m)"=w509:sgl, "height (m)"=w508:sgl)
        n209 = Strip Path(path=w485) -> (stripped path=w518:path, name=w517:string)
        n210 = Get Date/Time In Seconds() -> (seconds since 1Jan1904=w481:timestamp)
        n211 = Bundle By Name(cluster=T7 {"up/down"=FALSE, "time/line"=0.0, "start time"=timestamp(0 s since 1904-01-01), "end time"=timestamp(0 s since 1904-01-01)} ("Scan param"), "up/down"=TRUE, "time/line"=sgl nan ("input 7"), "start time"=w522, "end time"=w481) -> (w521:T7)
        n212 = Bundle By Name(cluster=T5 {"center X"=0.0, "center Y"=0.0, "angle"=0.0, "width"=0.0, "height"=0.0, "# pixels"=0, "# lines"=0} ("Scanfield"), "center X"=w512, "center Y"=w511, "angle"=w510, "width"=w509, "height"=w508, "# lines"=w505, "# pixels"=w506) -> (w507:T5)
        n213 = Bundle("stripped path"=w518, "name"=w517) -> (w516:cluster{"stripped path":path, "name":string})  [unwired: 1 in]
        n214 = call <userlib>:"Save sxm File.vi"("Auto file naming? (T)"=FALSE, "Scanfield"=w507, "Scan param"=w521, "error in (no error)"=w515, "Channels data"=w525, "Channels config"=T6 [{"Name"="Z (m)", "Calibration"=1.0, "Offset"=0.0, "Channel index"=0}], "Filename control"=w516) -> ("error out"=w491:errorcluster)  [unwired: 2 in, 2 out]
        n215 = Strip Path(path=w485) -> (stripped path=w495:path)  [unwired: 1 out]
        n216 = Strip Path(path=w495) -> (stripped path=w494:path)  [unwired: 1 out]
        n217 = call <userlib>:"Get Session Path.vi"("error in (no error)"=w491, "Application ref in"=w490) -> ("error out"=w487:errorcluster, "Session path"=w489:path, "Application ref out"=w474:refnum<vi>)  [unwired: 7 in]
        n218 = Path To String(path=w485) -> (string=w484:string)
        n219 = Path To String(path=w494) -> (string=w492:string)
        n220 = call "SXM.vi"("Path"=w489, "Delete"=FALSE, "error in"=w487) -> ("error out"=w486:errorcluster)  [unwired: 7 in]
        n221 = call "ChangeSessionV2.vi"("error in (no error)"=w486, "Session"=w492) -> ("error out"=w463:errorcluster)
        n222 = Format Date/Time String(time format string (%c)=" Finished at %y%m%d - %H%M%S ", seconds (now)=w481) -> (date/time string=w480:string)  [unwired: 1 in]
        n223 = local read "zFile"() -> (w461:refnum<file>)
        n224 = Close File(refnum=w461, error in=w463) -> (error out=w462:errorcluster)  [unwired: 1 out]
        n225 = Concatenate Strings(w484, "\r\n", w480) -> (w483:string)
        n226 = Search and Replace String(input string="Email when finished", search string="@") -> (number of replacements=w476:i32)  [unwired: 6 in, 3 out]
        n227 = Greater Than 0?(x=w476) -> (x > 0?=w475:bool)
        n228 = case shown="True" w475 {
          tunnel: w462 -> [_ w533]
          tunnel: w483 -> [_ w531]
          tunnel: "Email when finished" -> [_ w530]
          frame False {
          }
          frame True {
            n229 = call "Send Email"("error in"=w533, "Message"=w531, "Subject"="Grid Finished", "Recipients"=w530) -> ()  [unwired: 7 in, 1 out]
          }
        }
        n230 = local read "Imaging Bias"() -> (w464:dbl)
        n231 = call <userlib>:"BiasSpectroscopy SetProperties.vi"("Application ref in"=w474, "Z-Controller hold (no change)"=enum16{"no change", "on", "off"}."on") -> ("Application ref out"=w472:refnum<vi>)  [unwired: 12 in, 1 out]
        n232 = call <userlib>:"TipLift Set.vi"("TipLift (m)"=sgl 0.0, "Application ref in"=w472) -> ("Application ref out"=w469:refnum<vi>)  [unwired: 8 in, 1 out]
        n233 = call "move2mark (SubVI).vi"("Application in"=w469) -> ("Application out"=w465:refnum<vi>)  [unwired: 10 in]
        n234 = call <userlib>:"Voltage Set.vi"("Bias (V)"=w464, "Application ref in"=w465) -> ("Application ref out"=w466:refnum<vi>)  [unwired: 8 in, 1 out]
        n235 = call <userlib>:"Ctrl-on_off Set.vi"("Z Controller ON/OFF"=TRUE, "Application ref in"=w466) -> ("Application ref out"=w468:refnum<vi>)  [unwired: 8 in, 1 out]
        n236 = call <userlib>:"Point Erase.vi"("Application ref in"=w468, "Point index (-1=All points)"=-1) -> ("Application ref out"=w459:refnum<vi>)  [unwired: 12 in, 1 out]
        n237 = call "PLL_On_Off (SubVI).vi"("Output ON/OFF (F=OFF)"=FALSE, "Application in"=w459) -> ("Application out"=w460:refnum<vi>)  [unwired: 8 in, 1 out]
      }
    }
    "Error out" <- w42
    "Points taken" <- w10
    "X Offset" <- w9
    "Y Offset" <- w8
  }
